vi "File Start.vi"(5 "Run in Background":bool=TRUE, 7 "Write Period":u32=3000, 8 "Error In":errorcluster) -> (0 "Error Out":errorcluster)   [LabVIEW 2025, in "LOGlib_LV2025.lvlib"]
doc: "Starts writing logging statements to the default log file."
uses:
  LOGlib_LV2025.lvlib
  Support/File/Action.ctl
  File Run.vi
  Support/File/File.lvlib
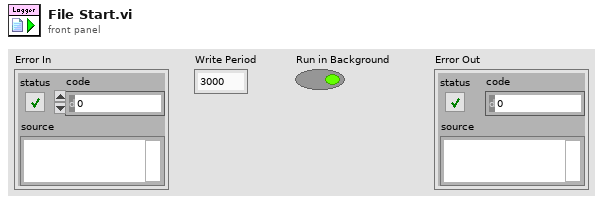
[diagram p1: front panel]
types:
  T1 = typedef "LOGlib_LV2025.lvlib/File.lvlib/Action.ctl" = enum16{"Initialize", "Set Maximum File Size", "Set Maximum File Count", "Set Root Folder", "Set Enable Calendar Folder Tree", "Set File Extension", "Set Prune All", "Set Delimiter", "Start", "Write", "Stop", "Shutdown"}
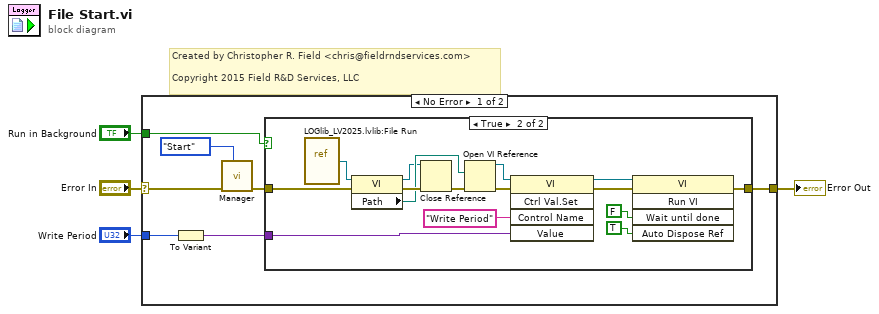
[diagram p0: block diagram]
diagram:
  # "Created by Christopher R. Field <chris@fieldrndservices.com>\n\nCopyright 2015 Field R&D Services, LLC"
  n1 = case shown="No Error" "Error In" {
    selector: "Error In" -> [w7 w28]
    tunnel: [w11 w28] -> w3
    tunnel: "Write Period" -> [w10 _]
    tunnel: "Run in Background" -> [w8 _]
    frame No Error {
      n2 = To Variant(anything=w10) -> (Variant=w9:variant)
      n3 = call "Manager.vi"("Action"=Action."Start", "Error In"=w7) -> ("Error Out"=w6:errorcluster)  [unwired: 9 in]
      n4 = case shown="True" w8 {
        tunnel: [w12 w20] -> w11
        tunnel: w9 -> [_ w14]
        tunnel: w6 -> [w12 w13]
        frame False {
        }
        frame True {
          n5 = vi-ref "LOGlib_LV2025.lvlib:File Run.vi"() -> (w25:refnum<vi>)
          n6 = property class="VI"(reference=w25, error in=w13) -> (reference out=w21:refnum<vi>, error out=w27:errorcluster, "Path"=w26:path)
          n7 = Close Reference(reference=w21, error in (no error)=w27) -> (error out=w22:errorcluster)
          n8 = Open VI Reference(vi path=w26, error in (no error)=w22) -> (vi reference=w19:refnum<vi>, error out=w17:errorcluster)  [unwired: 4 in]
          n9 = invoke class="VI" method="Ctrl Val.Set"(reference=w19, error in=w17, "Control Name"="Write Period", "Value"=w14) -> (reference out=w18:refnum<vi>, error out=w16:errorcluster)  [unwired: 1 in, 3 out]
          n10 = invoke class="VI" method="Run VI"(reference=w18, error in=w16, "Wait until done"=FALSE ("Wait Until Done"), "Auto Dispose Ref"=TRUE ("Auto Dispose Reference")) -> (error out=w20:errorcluster)  [unwired: 1 in, 4 out]
        }
      }
    }
    frame Error {
    }
  }
  "Error Out" <- w3
